vi "Real QR Factorization.vi"(0 "A":T1, 1 "algorithm":enum32{"Householder", "Givens", "Fast Givens"}(ring)) -> (2 "Q":T1, 3 "R":T1, 4 "error":i32)   [LabVIEW 2020, in "NI_AALPro.lvlib"]
doc: "Performs the QR factorization of <B> A</B>. You can use this polymorphic VI to perform QR factorization on a real matrix or a complex matrix. The data type you wire to the <B>A</B> input determines the polymorphic instance to use."
uses:
  <vilib>/Analysis/NI_AALPro.lvlib
  <vilib>/Analysis/Matrix/Datatypes/RealMatrix.ctl
  <resource>/lvanlys.dll
  <vilib>/Analysis/Matrix/NI_Matrix.lvlib
panel:
  # "QR Factorization"
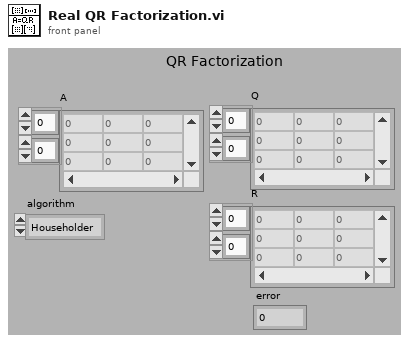
[diagram p1: front panel]
types:
  T1 = typedef "NI_Matrix.lvlib/RealMatrix.ctl" = dbl[][]
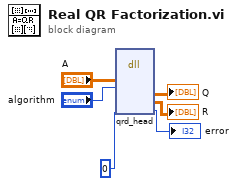
[diagram p0: block diagram]
diagram:
  n1 = dll-call lib="e:/builds/penguin/labview/branches/2020/dev/dist/resource/lvanlys.*" fn="qrd_head"("A"="A", "algorithm"="algorithm", 0) -> ("Q"=→"Q":T1, "R"=→"R":T1, →"error":i32)  [unwired: 8 in, 2 out]
